vi "Actor Core.vi"(8 "error in":errorcluster, 11 "Data Viewer in":refnum<class "Logging.lvclass">) -> (0 "error out":errorcluster, 3 "Actor out":refnum<class "Actor.lvclass">)   [LabVIEW 2020, in "Logging.lvlib" / "Logging.lvclass"]
doc: "The user interface for this panel.\n----\nCopyright: MGI 2016\nAuthor: Derek Trepanier"
uses:
  Logging.lvclass
  C:/Program Files/National Instruments/LabVIEW 2020/vi.lib/MGI/Panel Manager/Panel Actor/Panel Actor/Panel Actor.lvclass
  <vilib>/ActorFramework/Actor/Actor.lvclass
  <vilib>/ActorFramework/Message Enqueuer/Message Enqueuer.lvclass/Message Enqueuer.ctl
  <vilib>/ActorFramework/Message Enqueuer/Enqueue.vi
  <vilib>/ActorFramework/Stop Msg/Stop Msg.lvclass
  C:/Program Files/National Instruments/LabVIEW 2020/vi.lib/ActorFramework/Message/Message.lvclass
  <vilib>/ActorFramework/Message Priority Queue/Priority Enqueue.vi
  <vilib>/MGI/Panel Manager/Panel Actor/Panel Actor/Panel Actor.lvclass
  C:/Program Files/National Instruments/LabVIEW 2020/vi.lib/MGI/Monitored Actor/Monitored Actor/Monitored Actor/Monitored Actor.lvclass
  C:/Program Files/National Instruments/LabVIEW 2020/vi.lib/ActorFramework/Actor/Actor.lvclass
  \\coe-fs.engr.tamu.edu\Grads/renee.woodruff/Documents/LabVIEW Data/Bimanual Coord DAQ/Logging/Logging.lvclass
panel:
  # "Drag dataset(s) onto me"
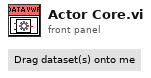
[diagram p1: front panel]
types:
  T1 = cluster{"Event Registration Refnum":refnum<event-registration>, "Pnl Actor":refnum<event-registration>}
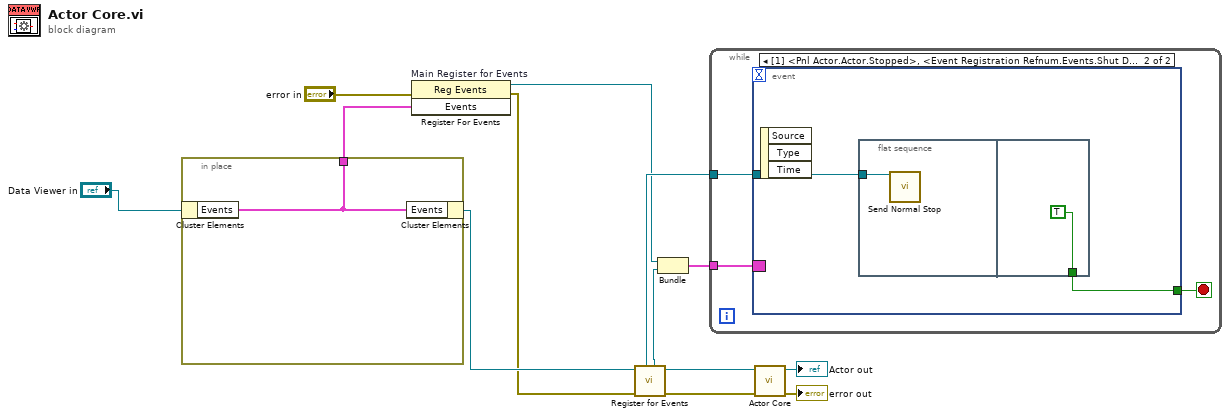
[diagram p0: block diagram]
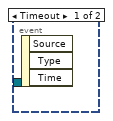
[diagram p2: hidden frame]
diagram:
  n1 = in-place {
    in-place-border: [w14] -> w5
    n2 = in-place-cluster #1("Data Viewer in") -> ("Events"=w14:cluster{"Shut Down":refnum<user-event>})
    n3 = in-place-cluster #1("Events"=w14) -> (w7:refnum<class "Logging.lvclass">)
  }
  n4 = register-events "Main Register for Events"(error in="error in", w5) -> (reference out=w2:refnum<event-registration>, error out=w4:errorcluster)  [unwired: 1 in]
  n5 = call <vilib>:"Register for Events.vi"("Error In"=w4, "Panel Actor in"=w7) -> ("Error Out"=w11:errorcluster, "Panel Actor out"=w10:refnum<class "Logging.lvclass">, "Pnl Actor"=w3:refnum<event-registration>, "Self Enqueuer"=w9:refnum<class "Message Enqueuer.lvclass">)  [unwired: 6 in]
  n6 = Bundle("Event Registration Refnum"=w2, "Pnl Actor"=w3) -> (w1:T1)  [unwired: 1 in]
  n7 = while {
    tunnel: w9 -> [w16]
    tunnel: w1 -> [w15]
    stop <- w17 stop-if-true
    n8 = event shown="[1] <Pnl Actor.Actor.Stopped>, <Event Registration Refnum.Events.Shut Down>: User Event" {
      selector: w15 -> [_ _]
      dyn-events: _ -> [_ _]
      timeout: _ -> [_ _]
      tunnel: [_ w19] -> w17
      tunnel: w16 -> [_ w18]
      event Timeout {
        n9 = event-data() -> ()  [unwired: 1 in, 3 out]
      }
      event User Event {
        n10 = event-data() -> ()  [unwired: 1 in, 3 out]
        n11 = flat-sequence {
          tunnel: w18 -> [w20]
          tunnel: [TRUE] -> w19
          frame #0 {
            n12 = call <vilib>:"Send Normal Stop.vi"("Message Enqueuer"=w20) -> ()  [unwired: 10 in, 1 out]
          }
          frame #1 {
          }
        }
      }
    }
  }
  n13 = call-parent "Actor Core.vi"("error in"=w11, "Panel Actor in"=w10) -> ("error out"=→"error out":errorcluster, "Actor out"=→"Actor out":refnum<class "Actor.lvclass">)  [unwired: 8 in]
